vi "koef coffeannan.vi"() -> ()   [LabVIEW 2020]
panel:
  in  "Tab Control":enum32{"Page 1", "Page 3", "Page 2"}(tab)
  out "Waveform Graph":dbl[][](graph)
  out "Waveform Graph 2":dbl[][](graph)
  out "Waveform Graph 3":dbl[][](graph)
  out "Waveform Graph 4":dbl[][](graph)
  out "Waveform Graph 8":dbl[][](graph)
  out "Waveform Graph 7":dbl[][](graph)
  out "Waveform Graph 6":dbl[][](graph)
  out "Waveform Graph 5":dbl[][](graph)
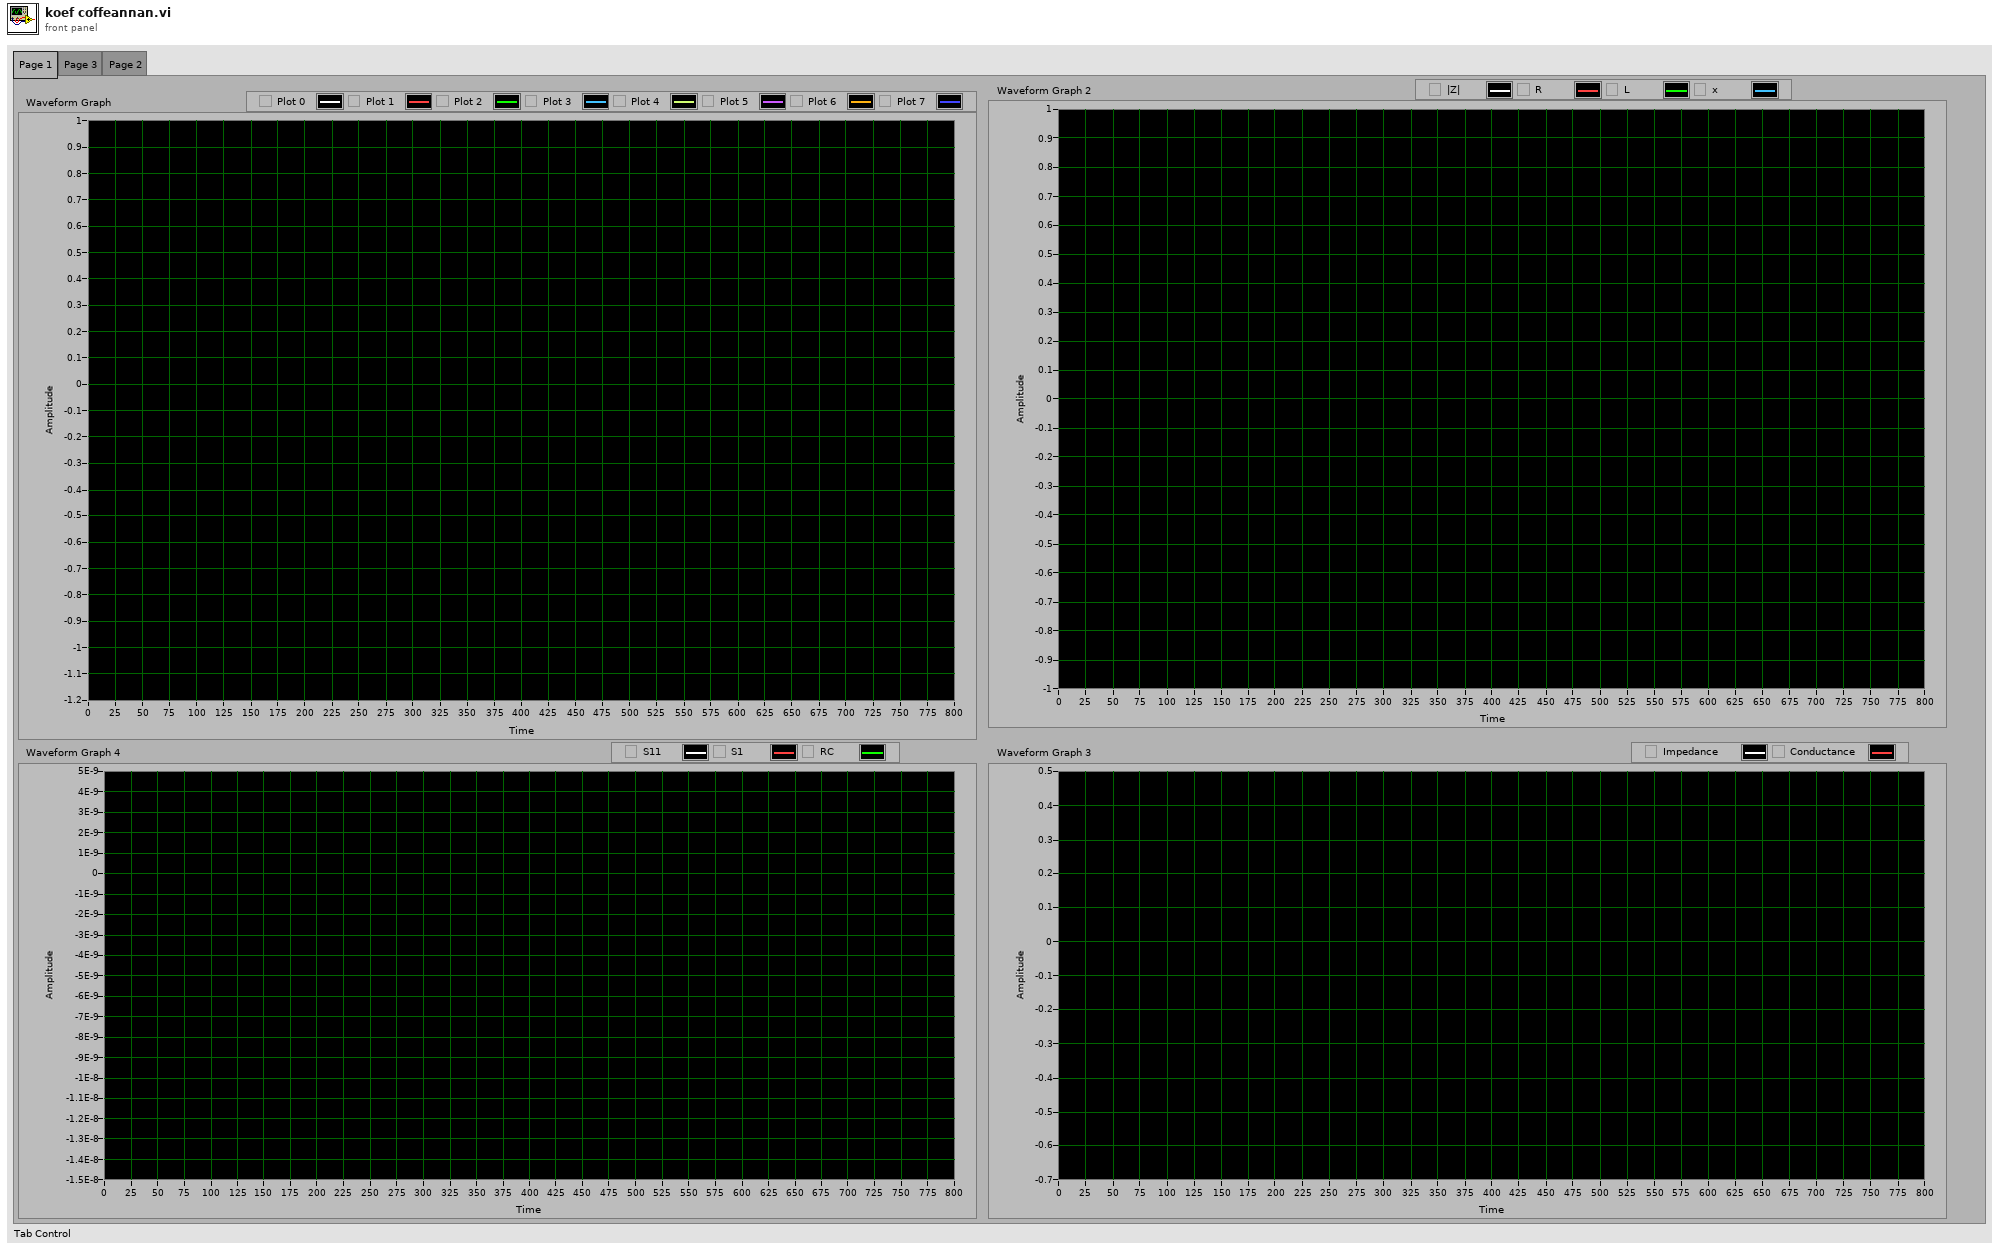
[diagram p1: front panel]
types:
  T1 = typedef "VFH-VNA_File_Handler.lvlib/VFH-file_cluster-Expensive.ctl" = cluster{"Frequency":dbl[], "Permativity'":dbl[], "Permativity''":dbl[], "Q [S/m]":dbl[], "Tan":dbl[], "Reflection R":dbl[], "Reflection I":dbl[]}
  T2 = typedef "VFH-VNA_File_Handler.lvlib/VFH-file_cluster-LabVIEWVNA.ctl" = cluster{"Frequency":dbl[], "S1_Real":dbl[], "S1_Imag":dbl[], "S11_Real":dbl[], "S11_Imag":dbl[], "S21_Real":dbl[], "S21_Imag":dbl[]}
  T3 = typedef "VFH-VNA_File_Handler.lvlib/VFH-file_cluster-NanoVNA.ctl" = cluster{"Frequency":dbl[], "S11_Real":dbl[], "S11_Imag":dbl[], "S21_Real":dbl[], "S21_Imag":dbl[], "S12_Real":dbl[], "S12_Imag":dbl[], "S22_Real":dbl[], "S22_Imag":dbl[]}
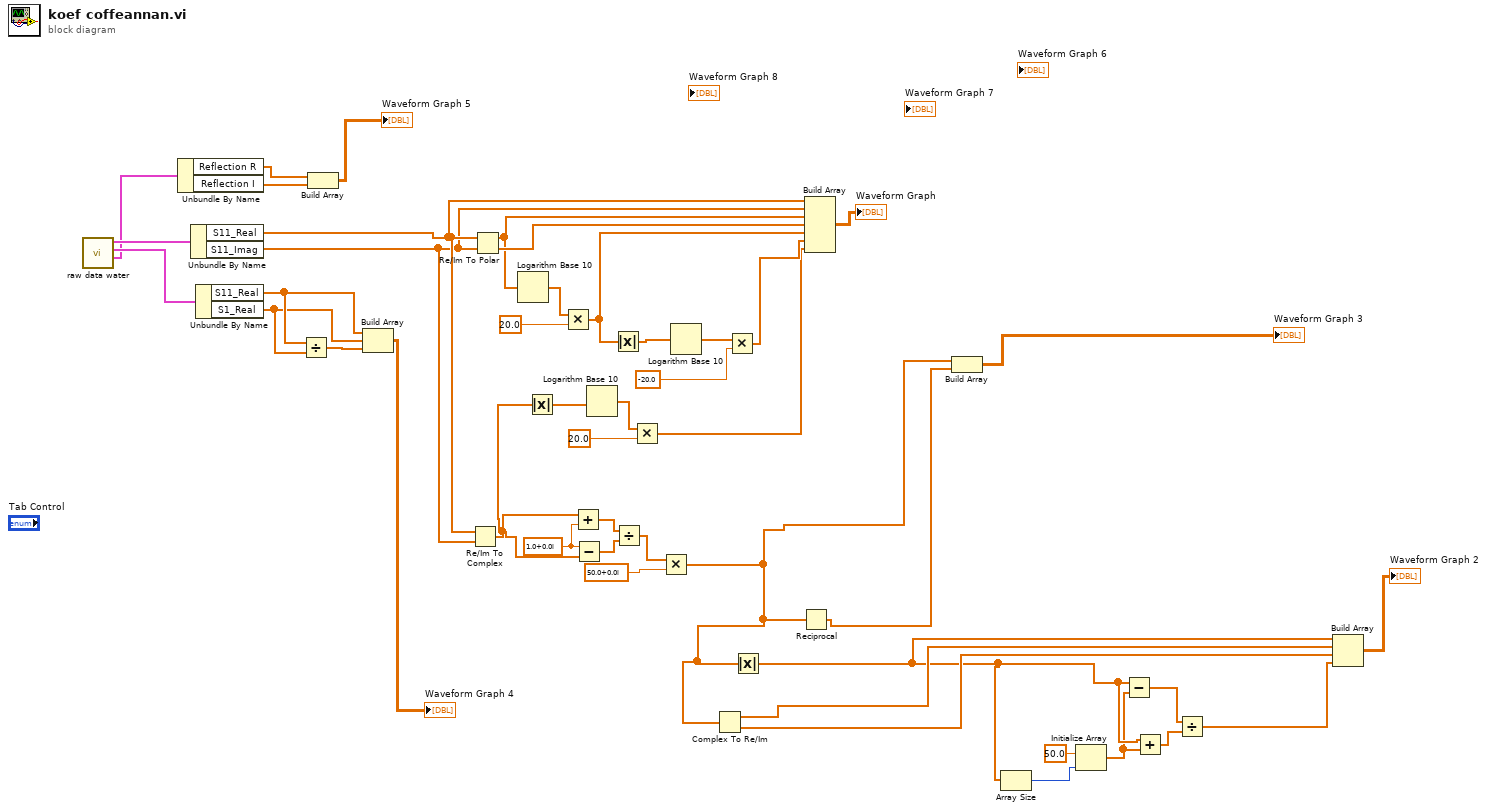
[diagram p0: block diagram]
diagram:
  w39 = cdb 1.0+0.0i ("x")
  n1 = call "raw data water.vi"() -> ("output R140"=w5:T1, "avg output LV"=w22:T2, "avg output NV"=w45:T3)  [unwired: 9 in]
  n2 = Unbundle By Name(w5) -> ("Reflection R"=w4:dbl[], "Reflection I"=w3:dbl[])
  n3 = Unbundle By Name(w45) -> ("S11_Real"=w34:dbl[], "S11_Imag"=w33:dbl[])
  n4 = Unbundle By Name(w22) -> ("S11_Real"=w21:dbl[], "S1_Real"=w20:dbl[])
  n5 = Divide(x=w21, y=w20) -> (x/y=w19:dbl[])
  n6 = Build Array(w4, w3) -> (→"Waveform Graph 5":dbl[][])
  n7 = Build Array(w21, w20, w19) -> (→"Waveform Graph 4":dbl[][])
  n8 = Re/Im To Complex(1:w33, 2:w34) -> (0:w8:cdb[])
  n9 = Re/Im To Polar(2:w33, 3:w34) -> (0:w44:dbl[], 1:w40:dbl[])
  n10 = Logarithm Base 10(1:w40) -> (0:w42:dbl[])
  n11 = Absolute Value(x=w8) -> (abs(x)=w7:dbl[])
  n12 = Multiply(x=w42, y=20.0) -> (x*y=w27:dbl[])
  n13 = Add(x=w8, y=w39) -> (x+y=w38:cdb[])
  n14 = Subtract(x=w39, y=w8) -> (x-y=w37:cdb[])
  n15 = Logarithm Base 10(1:w7) -> (0:w9:dbl[])
  n16 = Absolute Value(x=w27) -> (abs(x)=w26:dbl[])
  n17 = Divide(x=w38, y=w37) -> (x/y=w36:cdb[])
  n18 = Multiply(x=w9, y=20.0) -> (x*y=w6:dbl[])
  n19 = Multiply(x=w36, y=cdb 50.0+0.0i) -> (x*y=w28:cdb[])
  n20 = Logarithm Base 10(1:w26) -> (0:w25:dbl[])
  n21 = Complex To Re/Im(x + iy=w28) -> (x=w32:dbl[], y=w31:dbl[])
  n22 = Multiply(x=w25, y=-20.0) -> (x*y=w23:dbl[])
  n23 = Absolute Value(x=w28) -> (abs(x)=w15:dbl[])
  n24 = Reciprocal(x=w28) -> (1/x=w1:cdb[])
  n25 = Build Array(w34, w33, w40, w44, w27, w23, w6) -> (→"Waveform Graph":dbl[][])
  n26 = Build Array(w28, w1) -> (→"Waveform Graph 3":cdb[][])
  n27 = Array Size(array=w15) -> (size(s)=w16:i32)
  n28 = Initialize Array(50.0 ("element"), w16) -> (w14:dbl[])
  n29 = Subtract(x=w15, y=w14) -> (x-y=w12:dbl[])
  n30 = Add(x=w15, y=w14) -> (x+y=w13:dbl[])
  n31 = Divide(x=w12, y=w13) -> (x/y=w11:dbl[])
  n32 = Build Array(w15, w32, w31, w11) -> (→"Waveform Graph 2":dbl[][])
